vi "vTab_9234x2_CHx8.vi"() -> ()   [LabVIEW 2018]
uses:
  <vilib>/Utility/sysdir.llb/System Directory Type.ctl
  <vilib>/express/express analysis/Spectral/Block/exnSpectralBlock spectral measurements peak poly.vi
  <vilib>/express/express analysis/Spectral/Block/exnSpectralBlock spectral measurements peak DDT.vi
  <vilib>/ErrorRing/Error Ring.xnode
  <vilib>/express/express analysis/Spectral/XNode/ExpressSpectralMeasurementsBlockNode.xnode
  <vilib>/Utility/config.llb/NI_LVConfig.lvlib
panel:
  out "SVING":bool caption="存檔"
  in  "Open Folder":bool
  in  "Enable Saving":bool
  in  "Status":bool
  out "DA":bool caption="觸發"
  out "Time":timestamp format="%<%Y/%m/%d   %H:%M:%S>T"
  in  "Tab Control":enum32{"觸發訊號-C1", "觸發訊號-C2", "參數設定"}(tab)
  out "CH3-FFT":dynamicdata(graph)
  out "CH3-Timedomain":dynamicdata(graph)
  out "CH2-FFT":dynamicdata(graph)
  out "CH1-FFT":dynamicdata(graph)
  out "CH0-FFT":dynamicdata(graph)
  out "CH2-Timedomain":dynamicdata(graph)
  out "CH1-Timedomain":dynamicdata(graph)
  out "CH0-Timedomain":dynamicdata(graph)
  out "CH3-FFT":dynamicdata(graph)
  out "CH3-Timedomain":dynamicdata(graph)
  out "CH2-FFT":dynamicdata(graph)
  out "CH1-FFT":dynamicdata(graph)
  out "CH0-FFT":dynamicdata(graph)
  out "CH2-Timedomain":dynamicdata(graph)
  out "CH1-Timedomain":dynamicdata(graph)
  out "CH0-Timedomain":dynamicdata(graph)
  in  "Channel Selector (C1-C2)":bool[](array[boolean])=[TRUE, TRUE, TRUE, TRUE, TRUE, TRUE, TRUE, TRUE]
  in  "Lower Cut-Off (Hz)":dbl=100.0
  in  "Pre Samples":i32
  in  "Trigger Level":dbl=0.1 format="%#_13g"
  in  "觸發軸":enum32{"Channel 1", "Channel 2", "Channel 3"}(ring)
  in  "ABORT":bool
  in  "Run":bool
  out "DAQ Stoped":bool
  out "DAQ Data":dynamicdata(graph)
  in  "PAUSE":bool
  out "DAQ Error":errorcluster
  out "DAQ (N)":i32
  out "Main (N)":i32
  out "Buffer in Queue":i32(slide) scale=0.0..100.0
  out "Processed":dynamicdata(graph)
  in  "Sample Rate":dbl=10000.0 format="%#_13g"
  in  "Samples to Read":i32=10000
  in  "Trigger Slope":enum16{"Falling Edge", "Rising Edge"}(ring)=enum."Rising Edge"
  # "本頁畫面顯示為 觸發後訊號"
  # "FFT Filter by useing High-pass with Lower Cut-Off (Hz)"
  # "本頁畫面顯示為 觸發後訊號"
  # "FFT Filter by useing High-pass with Lower Cut-Off (Hz)"
  # "擷取卡設定"
  # "(系統開啟後修改無效)"
  # "軟體觸發設定"
  # "(修改即套用)"
  # "ExpressVI 設定擷取卡x2"
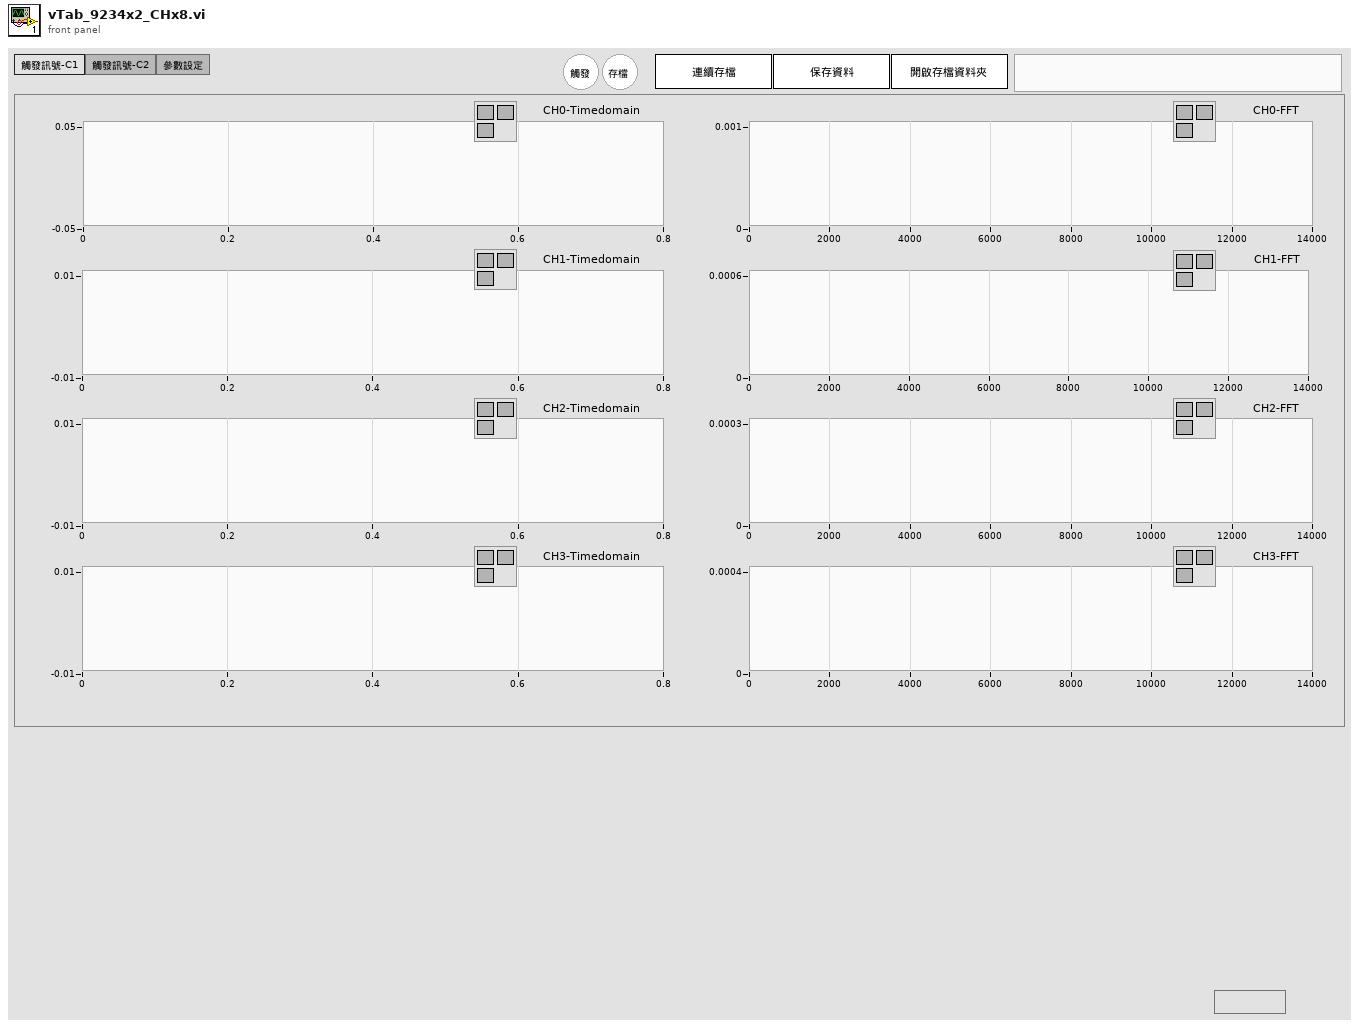
[diagram p1: front panel]
types:
  T1 = typedef "NI_LVConfig.lvlib/Config Data RefNum.ctl" = refnum<k1>
  T2 = enum8{"Enabled", "Disabled", "Disabled and Grayed Out"}
  T3 = cluster{"averaging mode":u16, "weighting mode":u16, "number of averages":u32}
  T4 = cluster{"dB On (F)":bool, "unwrap phase (F)":bool, "convert to degree (F)":bool}
  T5 = typedef "System Directory Type.ctl" = i32
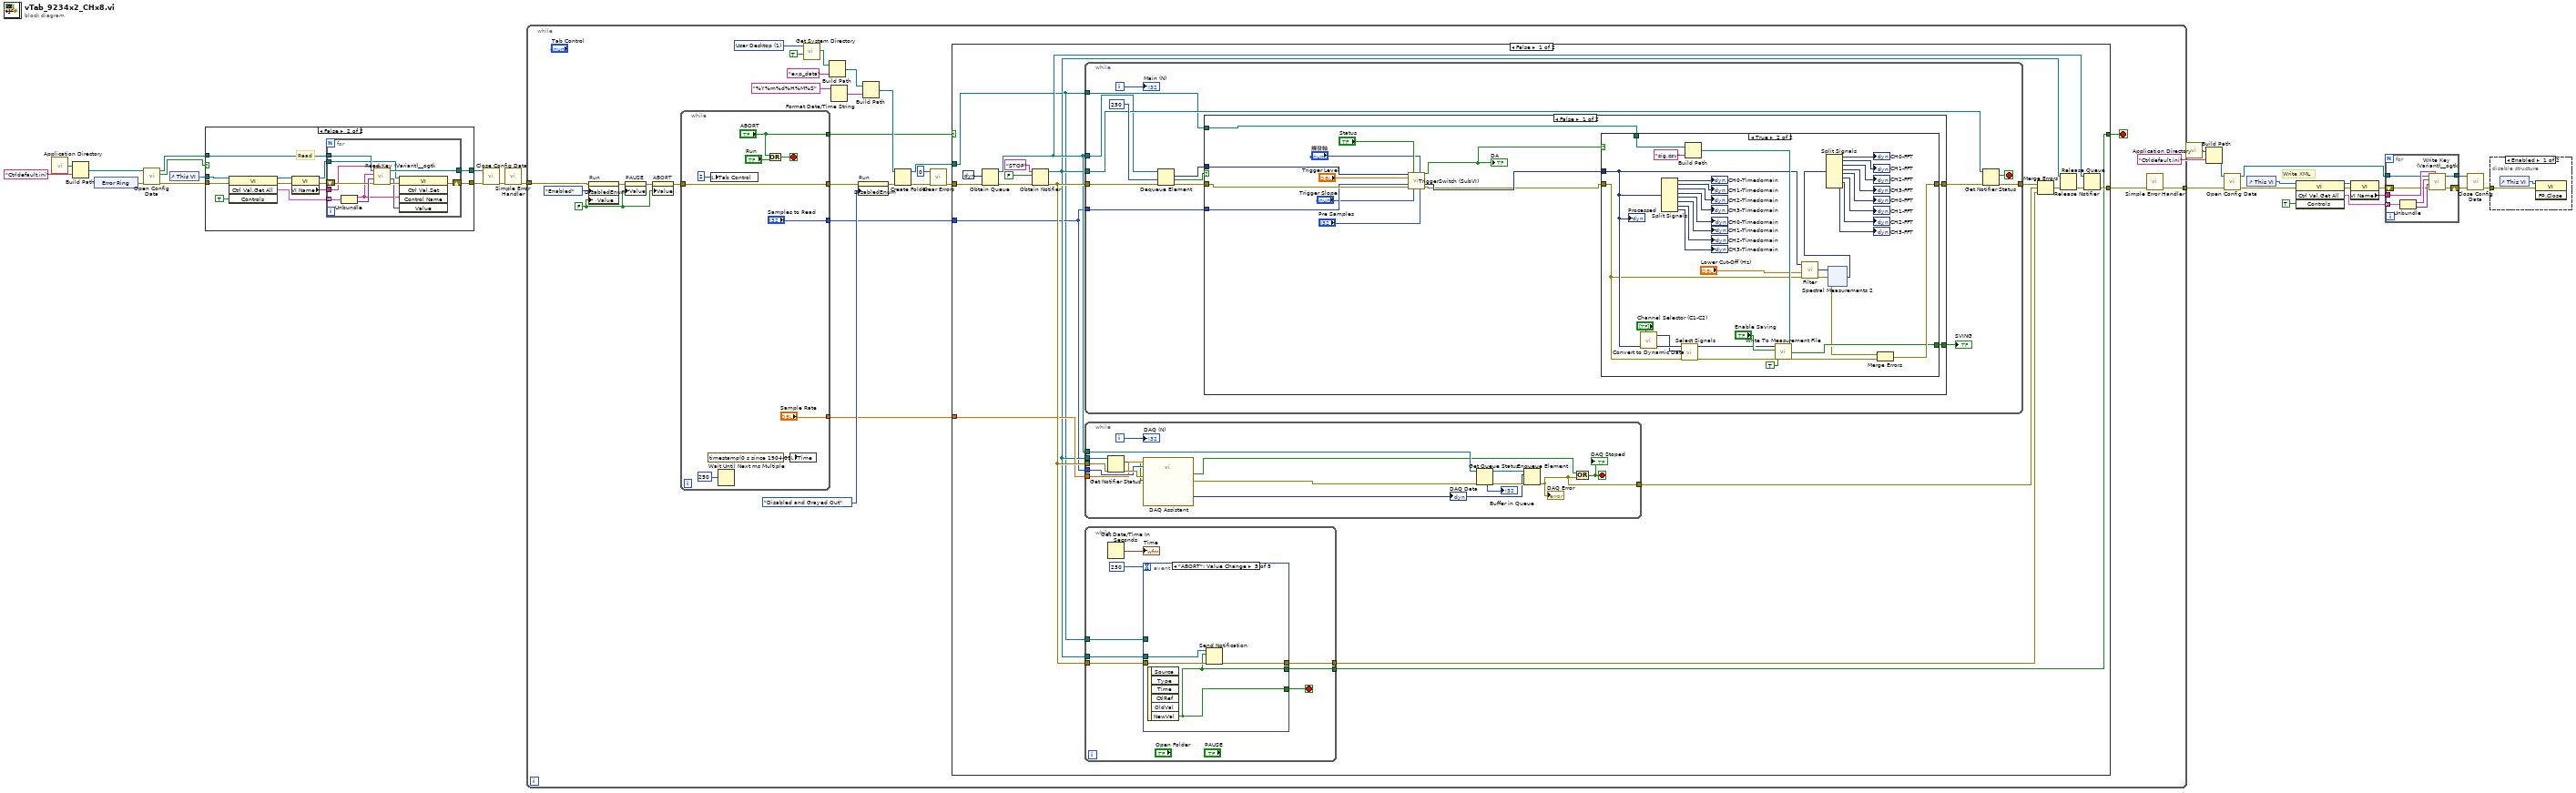
[diagram p0: block diagram]
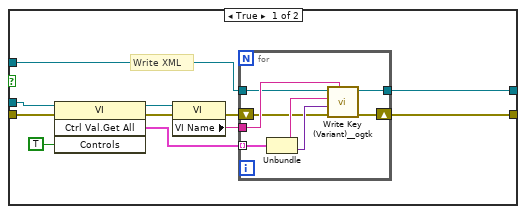
[diagram p2: hidden frame]
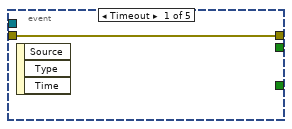
[diagram p6: hidden frame]
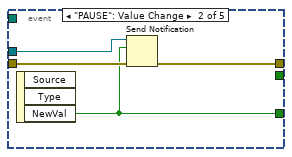
[diagram p7: hidden frame]
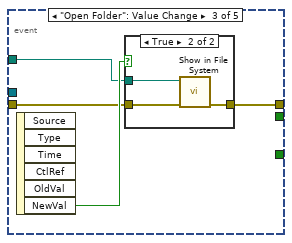
[diagram p8: hidden frame]
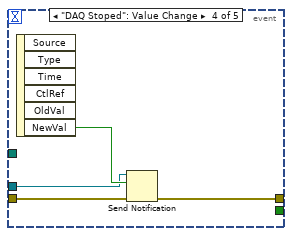
[diagram p10: hidden frame]
diagram:
  # "Write XML"
  n1 = call <vilib>:"Application Directory.vi"() -> ("Application Directory"=w1:path)
  n2 = Build Path(base path=w1, name or relative path="Ctrldefault.ini") -> (appended path=w28:path)
  n3 = xnode "Error Ring"() -> ("error out"=w20:errorcluster)
  n4 = call <vilib>:"Open Config Data.vi"("error in (no error)"=w20, "configuration file path"=w28) -> ("error out"=w25:errorcluster, "file created?"=w21:bool, "refnum"=w18:T1)  [unwired: 7 in]
  n5 = control-ref of="This VI"() -> (w19:refnum<vi>)
  n6 = case shown="False" w21 {
    tunnel: [w33 w53] -> w26
    tunnel: w25 -> [w31 w51]
    tunnel: [w29 w49] -> w24
    tunnel: w19 -> [w32 w52]
    tunnel: w18 -> [w34 w54]
    frame True {
      # "Write XML"
      n7 = invoke class="VI" method="Ctrl Val.Get All"(reference=w32, error in=w31, "Controls"=TRUE) -> (reference out=w38:refnum<vi>, error out=w37:errorcluster, "Get All Control Values Variant"=w39:cluster{"Name":string, "Variant Data":variant}[])  [unwired: 1 in, 1 out]
      n8 = property class="VI"(reference=w38, error in=w37) -> (error out=w30:errorcluster, "VI Name"=w36:string)  [unwired: 1 out]
      n9 = for {
        tunnel: w39 -> [w47] mode=indexing
        tunnel: w36 -> [w46]
        tunnel: w34 -> [w44]
        shift-right: [w43] -> w33
        shift-left: w30 -> [w41]
        tunnel: [w40] -> w29
        n10 = Unbundle(w47) -> ("Name"=w45:string, "Variant Data"=w42:variant)
        n11 = call <userlib>:"Write Key (Variant)__ogtk.vi"("section"=w46, "error in (no error)"=w41, "key-value"=w42, "key (optional)"=w45, "refnum"=w44) -> ("error out"=w43:errorcluster, "refnum out"=w40:T1)  [unwired: 5 in]
      }
    }
    frame False {
      # "Read"
      n12 = invoke class="VI" method="Ctrl Val.Get All"(reference=w52, error in=w51, "Controls"=TRUE) -> (reference out=w58:refnum<vi>, error out=w57:errorcluster, "Get All Control Values Variant"=w59:cluster{"Name":string, "Variant Data":variant}[])  [unwired: 1 in, 1 out]
      n13 = property class="VI"(reference=w58, error in=w57) -> (reference out=w48:refnum<vi>, error out=w50:errorcluster, "VI Name"=w56:string)
      n14 = for {
        tunnel: w59 -> [w70] mode=indexing
        tunnel: w56 -> [w63]
        tunnel: w54 -> [w69]
        shift-right: [w64] -> w53
        shift-left: w50 -> [w67]
        tunnel: [w66] -> w49
        tunnel: w48 -> [w62]
        n15 = Unbundle(w70) -> ("Name"=w60:string, "Variant Data"=w68:variant)
        n16 = call <userlib>:"Read Key (Variant)__ogtk.vi"("section"=w63, "error in (no error)"=w67, "type"=w68, "key (optional)"=w60, "refnum"=w69) -> ("error out"=w65:errorcluster, "key-value"=w61:variant, "refnum out"=w66:T1)  [unwired: 3 in, 1 out]
        n17 = invoke class="VI" method="Ctrl Val.Set"(reference=w62, error in=w65, "Control Name"=w60, "Value"=w61) -> (error out=w64:errorcluster)  [unwired: 1 in, 4 out]
      }
    }
  }
  n18 = call <vilib>:"Close Config Data.vi"("error in (no error)"=w26, "refnum"=w24) -> ("error out"=w23:errorcluster)  [unwired: 8 in, 1 out]
  n19 = call <vilib>:"Simple Error Handler.vi"("error in (no error)"=w23) -> ("error out"=w22:errorcluster)  [unwired: 4 in, 4 out]
  n20 = while {
    tunnel: [w97] -> w4
    tunnel: w22 -> [w73]
    stop <- w76 stop-if-true
    w86 = T5 1 items=["User Home"=0, "User Desktop"=1, "User Documents"=2, "User Application Data"=3, "User Preferences"=4, "User Temporary"=5, "Public Documents"=6, "Public Application Data"=7, "Public Preferences"=8, "Public Cache"=13, "System Core Libraries"=9, "System Installed Libraries"=10, "Application Files"=11, "Boot Volume Root"=12] ("system directory type")
    w91 = FALSE ("stop 3")
    n21 = property on="Run" class="Bool (strict)"(error in=w73, "DisabledEnum"=T2."Enabled" ("Disabled"), "Value"=w91) -> (error out=w94:errorcluster)  [unwired: 1 in, 1 out]
    n22 = property on="PAUSE" class="Bool (strict)"(error in=w94, "Value"=w91) -> (error out=w93:errorcluster)  [unwired: 1 in, 1 out]
    n23 = property on="ABORT" class="Bool (strict)"(error in=w93, "Value"=w91) -> (error out=w92:errorcluster)  [unwired: 1 in, 1 out]
    n24 = while {
      tunnel: [w246] -> w72
      tunnel: w92 -> [w246]
      tunnel: ["Samples to Read"] -> w75
      tunnel: ["Sample Rate"] -> w78
      tunnel: ["ABORT"] -> w71
      stop <- w240 stop-if-true
      n25 = local write "Tab Control"(2) -> ()
      n26 = Wait Until Next ms Multiple(millisecond multiple=u32 250) -> ()  [unwired: 1 out]
      n27 = Or(x="ABORT", y="Run") -> (x .or. y?=w240:bool)
      n28 = local write "Time"(timestamp(0 s since 1904-01-01) ("Time 2")) -> ()
    }
    n29 = call <vilib>:"Get System Directory.vi"("create directory if not found? (F)"=TRUE, "system directory type"=w86) -> ("system directory"=w88:path)  [unwired: 9 in]
    n30 = Build Path(base path=w88, name or relative path="exp_data") -> (appended path=w84:path)
    n31 = Format Date/Time String(time format string (%c)="%Y%m%d%H%M%S") -> (date/time string=w83:string)  [unwired: 2 in]
    n32 = property on="Run" class="Bool (strict)"(error in=w72, "DisabledEnum"=T2."Disabled and Grayed Out" ("Disabled")) -> (error out=w89:errorcluster)  [unwired: 1 in, 1 out]
    n33 = Build Path(base path=w84, name or relative path=w83) -> (appended path=w82:path)
    n34 = Create Folder(path (use dialog)=w82, error in=w89) -> (created path=w74:path, error out=w80:errorcluster)  [unwired: 1 in, 1 out]
    n35 = call <vilib>:"Clear Errors.vi"("error in (no error)"=w80, "specific error code to clear (0: all)"=0) -> ("error out"=w79:errorcluster)  [unwired: 4 in, 1 out]
    n36 = case shown="False" w71 {
      selector: w71 -> [_ w236]
      tunnel: w79 -> [w108 w237]
      tunnel: w78 -> [w107 _]
      tunnel: [w104 w237] -> w77
      tunnel: [w100 w236] -> w76
      tunnel: w75 -> [w99 _]
      tunnel: w74 -> [w98 _]
      frame False {
        n37 = Obtain Queue(element data type=dynamicdata [] ("data"), error in (no error)=w108) -> (queue out=w106:refnum<queue>, error out=w111:errorcluster)  [unwired: 3 in, 1 out]
        n38 = Obtain Notifier(name (unnamed)="STOP", notification data type=FALSE, error in (no error)=w111) -> (notifier out=w101:refnum<notifier>, error out=w114:errorcluster)  [unwired: 1 in, 1 out]
        n39 = while {
          tunnel: w106 -> [w120]
          tunnel: w114 -> [w127]
          tunnel: [w123] -> w102
          tunnel: w101 -> [w121]
          tunnel: w99 -> [w118]
          tunnel: w98 -> [w117]
          i -> [w129]
          stop <- w122 stop-if-true
          n40 = Dequeue Element(queue=w120, timeout in ms (-1)=250, error in (no error)=w127) -> (element=w126:dynamicdata, timed out?=w119:bool, error out=w125:errorcluster)  [unwired: 1 out]
          n41 = case shown="False" w119 {
            tunnel: w126 -> [w142 _]
            tunnel: w125 -> [w140 w190]
            tunnel: [w143 w190] -> w124
            tunnel: w118 -> [w137 _]
            tunnel: w117 -> [w136 _]
            tunnel: [w135 _] -> w116
            frame False {
              n42 = call "TriggerSwitch (SubVI).vi"("data"=w142, "TRIGGER SW"="Status", "Trigger Axis"="觸發軸", "Trigger Level"="Trigger Level", "Samples to Read"=w137, "error in (no error)"=w140, "Trigger Slope"="Trigger Slope", "Pre Samples"="Pre Samples") -> ("Data Available"=w130:bool, "Section"=w141:dynamicdata, "error out"=w139:errorcluster)  [unwired: 5 in]
              "DA" <- w130
              n43 = case shown="True" w130 {
                tunnel: w141 -> [_ w150]
                tunnel: w139 -> [w144 w147]
                tunnel: [w144 w173] -> w143
                tunnel: w136 -> [_ w170]
                tunnel: [_ w163] -> w135
                frame False {
                }
                frame True {
                  n44 = call "Convert to Dynamic Data"("Array"="Channel Selector (C1-C2)") -> ("Dynamic Data Type"=w148:dynamicdata)  [unwired: 3 in]
                  n45 = Split Signals(w150) -> (→"CH0-Timedomain":dynamicdata, →"CH1-Timedomain":dynamicdata, →"CH2-Timedomain":dynamicdata, →"CH3-Timedomain":dynamicdata, →"CH0-Timedomain":dynamicdata, →"CH1-Timedomain":dynamicdata, →"CH2-Timedomain":dynamicdata, →"CH3-Timedomain":dynamicdata)  [unwired: 8 in]
                  n46 = call "Select Signals"("error in (no error)"=w147, "Selector Input"=w148, "Signals"=w150) -> ("error out"=w146:errorcluster, "Signal Out"=w145:dynamicdata)  [unwired: 7 in]
                  n47 = Build Path(base path=w170, name or relative path="sig.csv") -> (appended path=w168:path)
                  n48 = call "Write To Measurement File"("Signals"=w145, "Enable"="Enable Saving", "new_file"=TRUE, "error in (no error)"=w146, "Filename"=w168) -> ("Saving Data"=w163:bool, "error out"=w151:errorcluster)  [unwired: 12 in, 1 out]
                  n49 = call "Filter"("error in (no error)"=w147, "Lower Cut-Off"="Lower Cut-Off (Hz)", "Signal"=w150) -> ("error out"=w166:errorcluster, "Filtered Signal"=w165:dynamicdata)  [unwired: 7 in]
                  n50 = xnode ("Spectral Measurements 2")("Signals"=w165, "error in (no error)"=w166) -> ("FFT - (Peak)"=w167:dynamicdata, "error out"=w162:errorcluster)  [unwired: 1 out]
                  n51 = Split Signals(w167) -> (→"CH0-FFT":dynamicdata, →"CH1-FFT":dynamicdata, →"CH2-FFT":dynamicdata, →"CH3-FFT":dynamicdata, →"CH0-FFT":dynamicdata, →"CH1-FFT":dynamicdata, →"CH2-FFT":dynamicdata, →"CH3-FFT":dynamicdata)  [unwired: 8 in]
                  n52 = Merge Errors(w162, w151) -> (w173:errorcluster)
                  "Processed" <- w150
                }
              }
            }
            frame True {
            }
          }
          "SVING" <- w116
          n53 = Get Notifier Status(notifier=w121, error in (no error)=w124) -> (current notification=w122:bool, error out=w123:errorcluster)  [unwired: 3 out]
          "Main (N)" <- w129
        }
        n54 = while {
          tunnel: w106 -> [w204]
          tunnel: [w196] -> w113
          tunnel: w114 -> [w200]
          tunnel: w101 -> [w198]
          tunnel: w99 -> [w195]
          tunnel: w107 -> [w194]
          i -> [w206]
          stop <- w197 stop-if-true
          n55 = Get Notifier Status(notifier=w198, error in (no error)=w200) -> (current notification=w193:bool, error out=w199:errorcluster)  [unwired: 3 out]
          n56 = call "DAQ Assistant"("rate"=w194, "number of samples"=w195, "error in"=w199, "stop (F)"=w193) -> ("data"=w191:dynamicdata, "stopped"=w192:bool, "error out"=w201:errorcluster)  [unwired: 12 in, 1 out]
          "DAQ Data" <- w191
          n57 = Get Queue Status(queue=w204, error in (no error)=w201) -> (queue out=w203:refnum<queue>, error out=w202:errorcluster, # elements in queue=→"Buffer in Queue":i32)  [unwired: 1 in, 5 out]
          n58 = Enqueue Element(queue=w203, element=w191, error in (no error)=w202) -> (error out=w196:errorcluster)  [unwired: 1 in, 2 out]
          "DAQ Error" <- w196
          n59 = Compound Arithmetic op=OR(w192, w196) -> (w197:bool)
          "DAQ Stoped" <- w197
          "DAQ (N)" <- w206
        }
        n60 = while {
          tunnel: w114 -> [w214]
          tunnel: [w213] -> w115
          tunnel: w101 -> [w211]
          tunnel: [w208] -> w100
          tunnel: w98 -> [w207]
          stop <- w209 stop-if-true
          n61 = Get Date/Time In Seconds() -> (seconds since 1Jan1904=→"Time":timestamp)
          n62 = event shown="[4] \"ABORT\": Value Change" {
            selector: _ -> [_ _ _ _ _]
            dyn-events: _ -> [_ _ _ _ _]
            timeout: 250 -> [_ _ _ _ _]
            tunnel: w214 -> [w215 w219 w222 w231 w235]
            tunnel: [w215 w218 w220 w228 w234] -> w213
            tunnel: w211 -> [_ w217 _ w229 w233]
            tunnel: [_ w216 _ _ w232] -> w209
            tunnel: [_ _ _ _ w232] -> w208
            tunnel: w207 -> [_ _ w221 _ _]
            event Timeout {
              n63 = event-data() -> ()  [unwired: 1 in, 3 out]
            }
            event "PAUSE": Value Change {
              n64 = event-data() -> ("NewVal"=w216:bool)  [unwired: 1 in, 2 out]
              n65 = Send Notification(notification=w216, notifier=w217, error in (no error)=w219) -> (error out=w218:errorcluster)  [unwired: 1 out]
            }
            event "Open Folder": Value Change {
              n66 = event-data() -> ("NewVal"=w223:bool)  [unwired: 1 in, 5 out]
              n67 = case shown="True" w223 {
                tunnel: w222 -> [w224 w227]
                tunnel: w221 -> [_ w226]
                tunnel: [w224 w225] -> w220
                frame False {
                }
                frame True {
                  n68 = call <vilib>:"Show in File System.vi"("error in (no error)"=w227, "file or directory path"=w226) -> ("error out"=w225:errorcluster)  [unwired: 9 in]
                }
              }
            }
            event "DAQ Stoped": Value Change {
              n69 = event-data() -> ("NewVal"=w230:bool)  [unwired: 1 in, 5 out]
              n70 = Send Notification(notification=w230, notifier=w229, error in (no error)=w231) -> (error out=w228:errorcluster)  [unwired: 1 out]
            }
            event "ABORT": Value Change {
              n71 = event-data() -> ("NewVal"=w232:bool)  [unwired: 1 in, 5 out]
              n72 = Send Notification(notification=w232, notifier=w233, error in (no error)=w235) -> (error out=w234:errorcluster)  [unwired: 1 out]
            }
          }
        }
        n73 = Merge Errors(w102, w113, w115) -> (w103:errorcluster)
        n74 = Release Notifier(notifier=w101, error in (no error)=w103) -> (error out=w105:errorcluster)  [unwired: 1 in, 2 out]
        n75 = Release Queue(queue=w106, error in (no error)=w105) -> (error out=w104:errorcluster)  [unwired: 1 in, 2 out]
      }
      frame True {
      }
    }
    n76 = call <vilib>:"Simple Error Handler.vi"("error in (no error)"=w77) -> ("error out"=w97:errorcluster)  [unwired: 4 in, 4 out]
  }
  n77 = call <vilib>:"Application Directory.vi"() -> ("Application Directory"=w2:path)
  n78 = Build Path(base path=w2, name or relative path="Ctrldefault.ini") -> (appended path=w11:path)
  n79 = call <vilib>:"Open Config Data.vi"("error in (no error)"=w4, "configuration file path"=w11) -> ("error out"=w14:errorcluster, "refnum"=w17:T1)  [unwired: 7 in, 1 out]
  n80 = control-ref of="This VI"() -> (w16:refnum<vi>)
  n81 = invoke class="VI" method="Ctrl Val.Get All"(reference=w16, error in=w14, "Controls"=TRUE) -> (reference out=w9:refnum<vi>, error out=w8:errorcluster, "Get All Control Values Variant"=w10:cluster{"Name":string, "Variant Data":variant}[])  [unwired: 1 in, 1 out]
  n82 = property class="VI"(reference=w9, error in=w8) -> (error out=w5:errorcluster, "VI Name"=w7:string)  [unwired: 1 out]
  n83 = for {
    tunnel: w10 -> [w254] mode=indexing
    tunnel: w7 -> [w253]
    tunnel: w17 -> [w251]
    shift-right: [w250] -> w13
    shift-left: w5 -> [w248]
    tunnel: [w247] -> w15
    n84 = Unbundle(w254) -> ("Name"=w252:string, "Variant Data"=w249:variant)
    n85 = call <userlib>:"Write Key (Variant)__ogtk.vi"("section"=w253, "error in (no error)"=w248, "key-value"=w249, "key (optional)"=w252, "refnum"=w251) -> ("error out"=w250:errorcluster, "refnum out"=w247:T1)  [unwired: 5 in]
  }
  n86 = call <vilib>:"Close Config Data.vi"("error in (no error)"=w13, "refnum"=w15) -> ("error out"=w3:errorcluster)  [unwired: 8 in, 1 out]
  n87 = disable-structure shown="Enabled" {
    disable-tunnel: w3 -> [w255 _]
    frame Enabled {
      n88 = control-ref of="This VI"() -> (w256:refnum<vi>)
      n89 = invoke class="VI" method="FP.Close"(reference=w256, error in=w255) -> ()  [unwired: 1 in, 3 out]
    }
    frame Disabled {
    }
  }
